vi "Initial_Autonomous.vi"() -> ()   [LabVIEW 2017]
uses:
  Destination.ctl
  Start Position.ctl
panel:
  in  "Start Position":T1
  in  "Destination":T2
  # "Initial Autonomous Mode FRC 2018"
  # "This program starts the initial autonomous mode for the FIRST Robotics Competition 2018. The operator selects the start position (A, B, C) and destination (1, 2, 3, 4) from the front panel, and the robot will navigate to the destination and drop off its block."
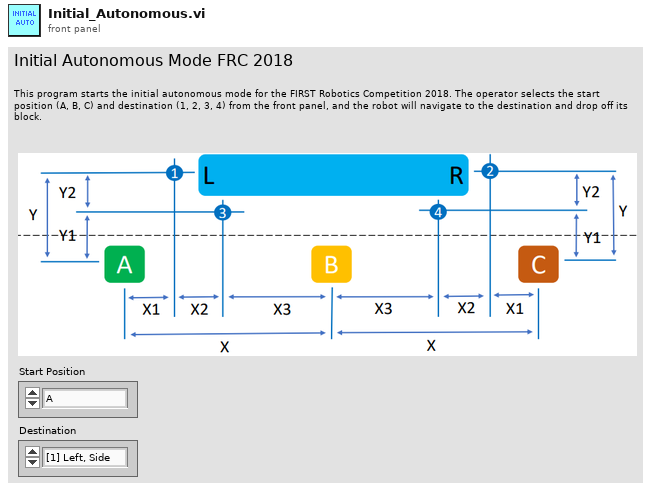
[diagram p1: front panel]
types:
  T1 = typedef "Start Position.ctl" = enum16{"A", "B", "C"}
  T2 = typedef "Destination.ctl" = enum16{"[1] Left, Side ", "[2] Right, Side", "[3] Left, Front", "[4] Right, Front"}
  T3 = typedef "Command Status Info.ctl" = cluster{"Name":string, "Status":T4, "notifier out":T5}
  T4 = typedef "Completion Status.ctl" = enum16{"Successful", "Aborted", "Incomplete"}
  T5 = typedef "Completion Notifier.ctl" = refnum<notifier>
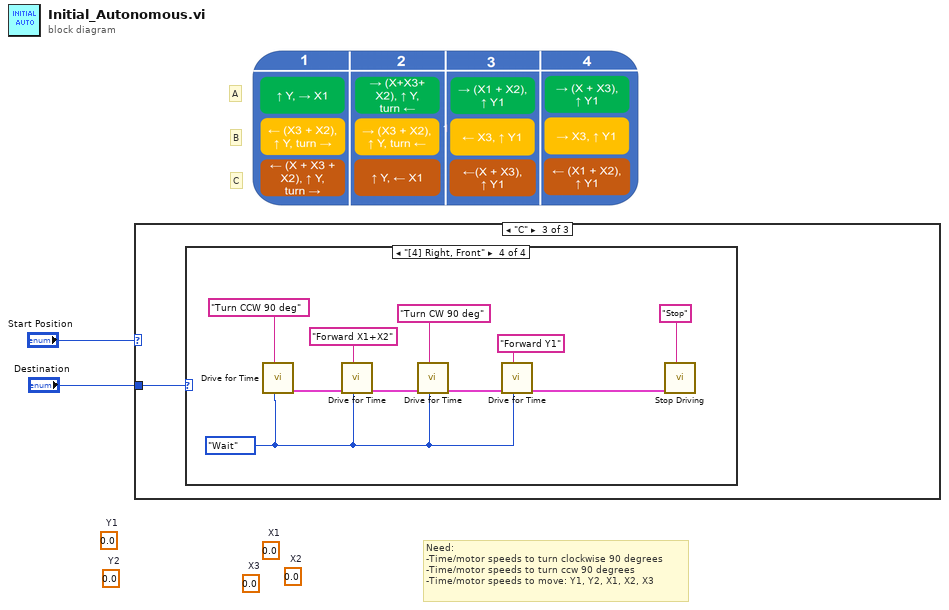
[diagram p0: block diagram]
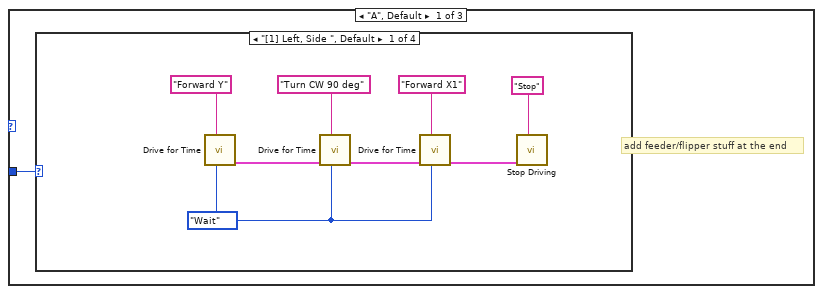
[diagram p2: hidden frame]
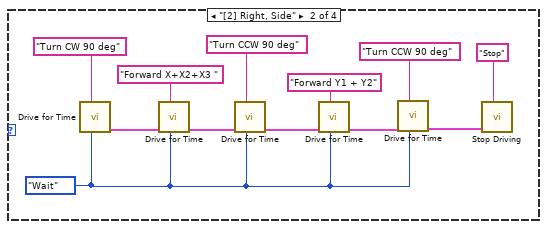
[diagram p3: hidden frame]
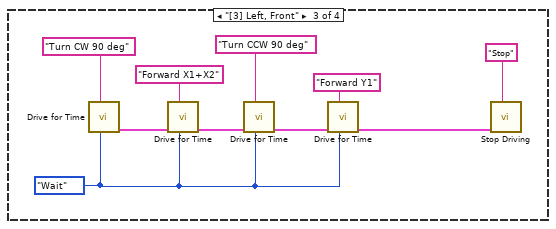
[diagram p4: hidden frame]
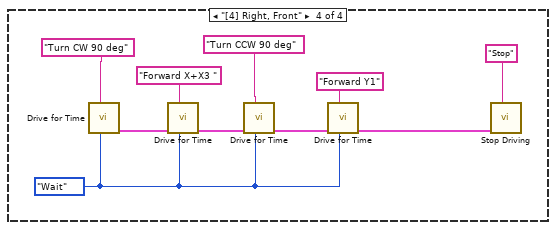
[diagram p5: hidden frame]
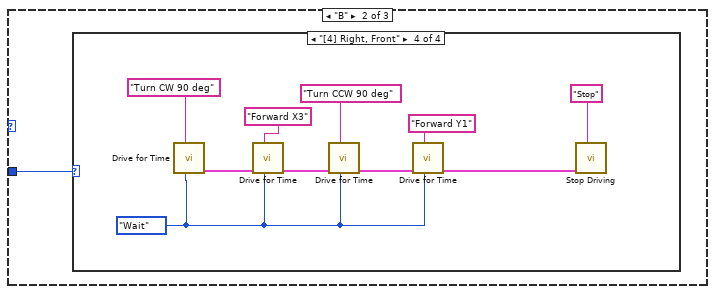
[diagram p6: hidden frame]
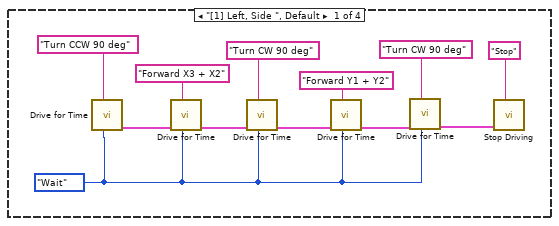
[diagram p7: hidden frame]
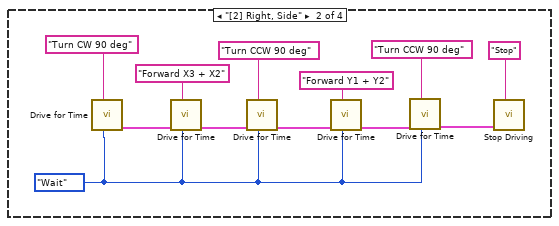
[diagram p8: hidden frame]
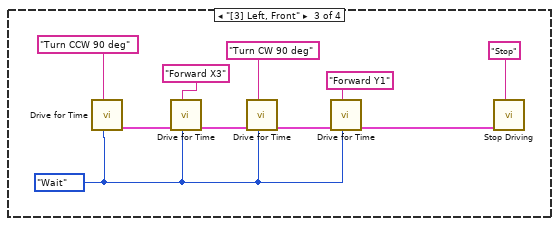
[diagram p9: hidden frame]
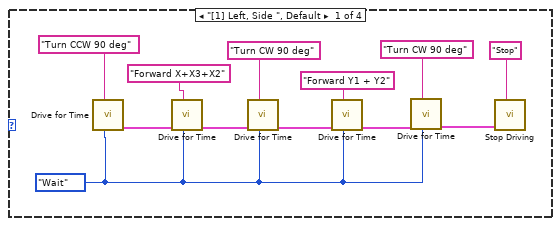
[diagram p10: hidden frame]
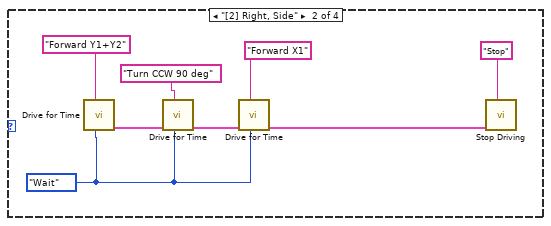
[diagram p11: hidden frame]
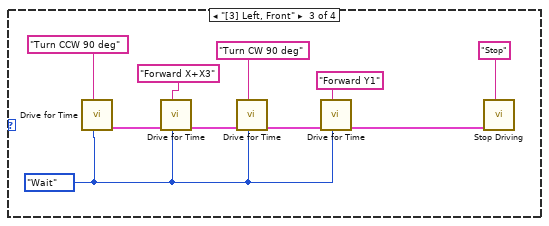
[diagram p12: hidden frame]
diagram:
  (unwired) 0.0  # X2
  (unwired) 0.0  # X1
  (unwired) 0.0  # X3
  (unwired) 0.0  # Y2
  (unwired) 0.0  # Y1
  # "Need:\n-Time/motor speeds to turn clockwise 90 degrees\n-Time/motor speeds to turn ccw 90 degrees\n-Time/motor speeds to move: Y1, Y2, X1, X2, X3"
  # "C"
  # "B"
  # "A"
  n1 = case shown="\"C\"" "Start Position" {
    tunnel: "Destination" -> [w3 w44 w89]
    frame "A", Default {
      # "add feeder/flipper stuff at the end"
      n2 = case shown="\"[1] Left, Side \", Default" w3 {
        frame "[1] Left, Side ", Default {
          w5 = enum16{"Start", "Wait"}."Wait" ("Synchronication")
          n3 = call "Drive for Time.vi"("Synchronization"=w5, "Description"="Forward Y") -> ("Command Info Out"=w11:T3)  [unwired: 8 in, 1 out]
          n4 = call "Drive for Time.vi"("Synchronization"=w5, "Description"="Turn CW 90 deg", "Command Info In"=w11) -> ("Command Info Out"=w7:T3)  [unwired: 7 in, 1 out]
          n5 = call "Drive for Time.vi"("Synchronization"=w5, "Description"="Forward X1", "Command Info In"=w7) -> ("Command Info Out"=w4:T3)  [unwired: 7 in, 1 out]
          n6 = call "Stop Driving.vi"("Description"="Stop", "Command Info In"=w4) -> ()  [unwired: 9 in, 1 out]
        }
        frame "[2] Right, Side" {
          w12 = enum16{"Start", "Wait"}."Wait" ("Synchronication")
          n7 = call "Drive for Time.vi"("Synchronization"=w12, "Description"="Turn CW 90 deg") -> ("Command Info Out"=w18:T3)  [unwired: 8 in, 1 out]
          n8 = call "Drive for Time.vi"("Synchronization"=w12, "Description"="Forward X+X2+X3 ", "Command Info In"=w18) -> ("Command Info Out"=w23:T3)  [unwired: 7 in, 1 out]
          n9 = call "Drive for Time.vi"("Synchronization"=w12, "Description"="Turn CCW 90 deg", "Command Info In"=w23) -> ("Command Info Out"=w16:T3)  [unwired: 7 in, 1 out]
          n10 = call "Drive for Time.vi"("Synchronization"=w12, "Description"="Forward Y1 + Y2", "Command Info In"=w16) -> ("Command Info Out"=w15:T3)  [unwired: 7 in, 1 out]
          n11 = call "Drive for Time.vi"("Synchronization"=w12, "Description"="Turn CCW 90 deg", "Command Info In"=w15) -> ("Command Info Out"=w14:T3)  [unwired: 7 in, 1 out]
          n12 = call "Stop Driving.vi"("Description"="Stop", "Command Info In"=w14) -> ()  [unwired: 9 in, 1 out]
        }
        frame "[3] Left, Front" {
          w25 = enum16{"Start", "Wait"}."Wait" ("Synchronication")
          n13 = call "Drive for Time.vi"("Synchronization"=w25, "Description"="Turn CW 90 deg") -> ("Command Info Out"=w28:T3)  [unwired: 8 in, 1 out]
          n14 = call "Drive for Time.vi"("Synchronization"=w25, "Description"="Forward X1+X2", "Command Info In"=w28) -> ("Command Info Out"=w33:T3)  [unwired: 7 in, 1 out]
          n15 = call "Drive for Time.vi"("Synchronization"=w25, "Description"="Turn CCW 90 deg", "Command Info In"=w33) -> ("Command Info Out"=w26:T3)  [unwired: 7 in, 1 out]
          n16 = call "Drive for Time.vi"("Synchronization"=w25, "Description"="Forward Y1", "Command Info In"=w26) -> ("Command Info Out"=w24:T3)  [unwired: 7 in, 1 out]
          n17 = call "Stop Driving.vi"("Description"="Stop", "Command Info In"=w24) -> ()  [unwired: 9 in, 1 out]
        }
        frame "[4] Right, Front" {
          w40 = enum16{"Start", "Wait"}."Wait" ("Synchronication")
          n18 = call "Drive for Time.vi"("Synchronization"=w40, "Description"="Turn CW 90 deg") -> ("Command Info Out"=w42:T3)  [unwired: 8 in, 1 out]
          n19 = call "Drive for Time.vi"("Synchronization"=w40, "Description"="Forward X+X3 ", "Command Info In"=w42) -> ("Command Info Out"=w41:T3)  [unwired: 7 in, 1 out]
          n20 = call "Drive for Time.vi"("Synchronization"=w40, "Description"="Turn CCW 90 deg", "Command Info In"=w41) -> ("Command Info Out"=w43:T3)  [unwired: 7 in, 1 out]
          n21 = call "Drive for Time.vi"("Synchronization"=w40, "Description"="Forward Y1", "Command Info In"=w43) -> ("Command Info Out"=w34:T3)  [unwired: 7 in, 1 out]
          n22 = call "Stop Driving.vi"("Description"="Stop", "Command Info In"=w34) -> ()  [unwired: 9 in, 1 out]
        }
      }
    }
    frame "B" {
      n23 = case shown="\"[4] Right, Front\"" w44 {
        frame "[1] Left, Side ", Default {
          w45 = enum16{"Start", "Wait"}."Wait" ("Synchronication")
          n24 = call "Drive for Time.vi"("Synchronization"=w45, "Description"="Turn CCW 90 deg") -> ("Command Info Out"=w51:T3)  [unwired: 8 in, 1 out]
          n25 = call "Drive for Time.vi"("Synchronization"=w45, "Description"="Forward X3 + X2", "Command Info In"=w51) -> ("Command Info Out"=w56:T3)  [unwired: 7 in, 1 out]
          n26 = call "Drive for Time.vi"("Synchronization"=w45, "Description"="Turn CW 90 deg", "Command Info In"=w56) -> ("Command Info Out"=w49:T3)  [unwired: 7 in, 1 out]
          n27 = call "Drive for Time.vi"("Synchronization"=w45, "Description"="Forward Y1 + Y2", "Command Info In"=w49) -> ("Command Info Out"=w48:T3)  [unwired: 7 in, 1 out]
          n28 = call "Drive for Time.vi"("Synchronization"=w45, "Description"="Turn CW 90 deg", "Command Info In"=w48) -> ("Command Info Out"=w47:T3)  [unwired: 7 in, 1 out]
          n29 = call "Stop Driving.vi"("Description"="Stop", "Command Info In"=w47) -> ()  [unwired: 9 in, 1 out]
        }
        frame "[2] Right, Side" {
          w57 = enum16{"Start", "Wait"}."Wait" ("Synchronication")
          n30 = call "Drive for Time.vi"("Synchronization"=w57, "Description"="Turn CW 90 deg") -> ("Command Info Out"=w63:T3)  [unwired: 8 in, 1 out]
          n31 = call "Drive for Time.vi"("Synchronization"=w57, "Description"="Forward X3 + X2", "Command Info In"=w63) -> ("Command Info Out"=w68:T3)  [unwired: 7 in, 1 out]
          n32 = call "Drive for Time.vi"("Synchronization"=w57, "Description"="Turn CCW 90 deg", "Command Info In"=w68) -> ("Command Info Out"=w61:T3)  [unwired: 7 in, 1 out]
          n33 = call "Drive for Time.vi"("Synchronization"=w57, "Description"="Forward Y1 + Y2", "Command Info In"=w61) -> ("Command Info Out"=w60:T3)  [unwired: 7 in, 1 out]
          n34 = call "Drive for Time.vi"("Synchronization"=w57, "Description"="Turn CCW 90 deg", "Command Info In"=w60) -> ("Command Info Out"=w59:T3)  [unwired: 7 in, 1 out]
          n35 = call "Stop Driving.vi"("Description"="Stop", "Command Info In"=w59) -> ()  [unwired: 9 in, 1 out]
        }
        frame "[3] Left, Front" {
          w70 = enum16{"Start", "Wait"}."Wait" ("Synchronication")
          n36 = call "Drive for Time.vi"("Synchronization"=w70, "Description"="Turn CCW 90 deg") -> ("Command Info Out"=w73:T3)  [unwired: 8 in, 1 out]
          n37 = call "Drive for Time.vi"("Synchronization"=w70, "Description"="Forward X3", "Command Info In"=w73) -> ("Command Info Out"=w78:T3)  [unwired: 7 in, 1 out]
          n38 = call "Drive for Time.vi"("Synchronization"=w70, "Description"="Turn CW 90 deg", "Command Info In"=w78) -> ("Command Info Out"=w71:T3)  [unwired: 7 in, 1 out]
          n39 = call "Drive for Time.vi"("Synchronization"=w70, "Description"="Forward Y1", "Command Info In"=w71) -> ("Command Info Out"=w69:T3)  [unwired: 7 in, 1 out]
          n40 = call "Stop Driving.vi"("Description"="Stop", "Command Info In"=w69) -> ()  [unwired: 9 in, 1 out]
        }
        frame "[4] Right, Front" {
          w80 = enum16{"Start", "Wait"}."Wait" ("Synchronication")
          n41 = call "Drive for Time.vi"("Synchronization"=w80, "Description"="Turn CW 90 deg") -> ("Command Info Out"=w83:T3)  [unwired: 8 in, 1 out]
          n42 = call "Drive for Time.vi"("Synchronization"=w80, "Description"="Forward X3", "Command Info In"=w83) -> ("Command Info Out"=w88:T3)  [unwired: 7 in, 1 out]
          n43 = call "Drive for Time.vi"("Synchronization"=w80, "Description"="Turn CCW 90 deg", "Command Info In"=w88) -> ("Command Info Out"=w81:T3)  [unwired: 7 in, 1 out]
          n44 = call "Drive for Time.vi"("Synchronization"=w80, "Description"="Forward Y1", "Command Info In"=w81) -> ("Command Info Out"=w79:T3)  [unwired: 7 in, 1 out]
          n45 = call "Stop Driving.vi"("Description"="Stop", "Command Info In"=w79) -> ()  [unwired: 9 in, 1 out]
        }
      }
    }
    frame "C" {
      n46 = case shown="\"[4] Right, Front\"" w89 {
        frame "[1] Left, Side ", Default {
          w90 = enum16{"Start", "Wait"}."Wait" ("Synchronication")
          n47 = call "Drive for Time.vi"("Synchronization"=w90, "Description"="Turn CCW 90 deg") -> ("Command Info Out"=w96:T3)  [unwired: 8 in, 1 out]
          n48 = call "Drive for Time.vi"("Synchronization"=w90, "Description"="Forward X+X3+X2", "Command Info In"=w96) -> ("Command Info Out"=w101:T3)  [unwired: 7 in, 1 out]
          n49 = call "Drive for Time.vi"("Synchronization"=w90, "Description"="Turn CW 90 deg", "Command Info In"=w101) -> ("Command Info Out"=w94:T3)  [unwired: 7 in, 1 out]
          n50 = call "Drive for Time.vi"("Synchronization"=w90, "Description"="Forward Y1 + Y2", "Command Info In"=w94) -> ("Command Info Out"=w93:T3)  [unwired: 7 in, 1 out]
          n51 = call "Drive for Time.vi"("Synchronization"=w90, "Description"="Turn CW 90 deg", "Command Info In"=w93) -> ("Command Info Out"=w92:T3)  [unwired: 7 in, 1 out]
          n52 = call "Stop Driving.vi"("Description"="Stop", "Command Info In"=w92) -> ()  [unwired: 9 in, 1 out]
        }
        frame "[2] Right, Side" {
          w103 = enum16{"Start", "Wait"}."Wait" ("Synchronication")
          n53 = call "Drive for Time.vi"("Synchronization"=w103, "Description"="Forward Y1+Y2") -> ("Command Info Out"=w105:T3)  [unwired: 8 in, 1 out]
          n54 = call "Drive for Time.vi"("Synchronization"=w103, "Description"="Turn CCW 90 deg", "Command Info In"=w105) -> ("Command Info Out"=w109:T3)  [unwired: 7 in, 1 out]
          n55 = call "Drive for Time.vi"("Synchronization"=w103, "Description"="Forward X1", "Command Info In"=w109) -> ("Command Info Out"=w102:T3)  [unwired: 7 in, 1 out]
          n56 = call "Stop Driving.vi"("Description"="Stop", "Command Info In"=w102) -> ()  [unwired: 9 in, 1 out]
        }
        frame "[3] Left, Front" {
          w111 = enum16{"Start", "Wait"}."Wait" ("Synchronication")
          n57 = call "Drive for Time.vi"("Synchronization"=w111, "Description"="Turn CCW 90 deg") -> ("Command Info Out"=w114:T3)  [unwired: 8 in, 1 out]
          n58 = call "Drive for Time.vi"("Synchronization"=w111, "Description"="Forward X+X3", "Command Info In"=w114) -> ("Command Info Out"=w119:T3)  [unwired: 7 in, 1 out]
          n59 = call "Drive for Time.vi"("Synchronization"=w111, "Description"="Turn CW 90 deg", "Command Info In"=w119) -> ("Command Info Out"=w112:T3)  [unwired: 7 in, 1 out]
          n60 = call "Drive for Time.vi"("Synchronization"=w111, "Description"="Forward Y1", "Command Info In"=w112) -> ("Command Info Out"=w110:T3)  [unwired: 7 in, 1 out]
          n61 = call "Stop Driving.vi"("Description"="Stop", "Command Info In"=w110) -> ()  [unwired: 9 in, 1 out]
        }
        frame "[4] Right, Front" {
          w121 = enum16{"Start", "Wait"}."Wait" ("Synchronication")
          n62 = call "Drive for Time.vi"("Synchronization"=w121, "Description"="Turn CCW 90 deg") -> ("Command Info Out"=w124:T3)  [unwired: 8 in, 1 out]
          n63 = call "Drive for Time.vi"("Synchronization"=w121, "Description"="Forward X1+X2", "Command Info In"=w124) -> ("Command Info Out"=w129:T3)  [unwired: 7 in, 1 out]
          n64 = call "Drive for Time.vi"("Synchronization"=w121, "Description"="Turn CW 90 deg", "Command Info In"=w129) -> ("Command Info Out"=w122:T3)  [unwired: 7 in, 1 out]
          n65 = call "Drive for Time.vi"("Synchronization"=w121, "Description"="Forward Y1", "Command Info In"=w122) -> ("Command Info Out"=w120:T3)  [unwired: 7 in, 1 out]
          n66 = call "Stop Driving.vi"("Description"="Stop", "Command Info In"=w120) -> ()  [unwired: 9 in, 1 out]
        }
      }
    }
  }
